vi "MoveToAndRotate.vi"(5 "Camera Offset Y":dbl, 6 "Initial Angle":dbl, 7 "Camera Offset X":dbl, 8 "Error In":errorcluster, 9 "Probing Array":dbl[][](array[numeric]), 10 "Probe Index":i32, 11 "connection ID":refnum<k5>) -> (0 "error out":errorcluster, 3 "connection ID 2":refnum<k5>)   [LabVIEW 2018]
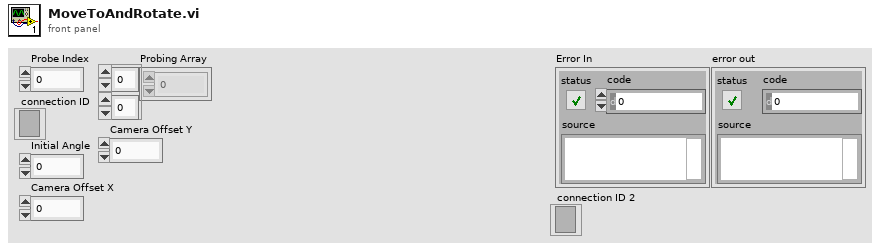
[diagram p1: front panel]
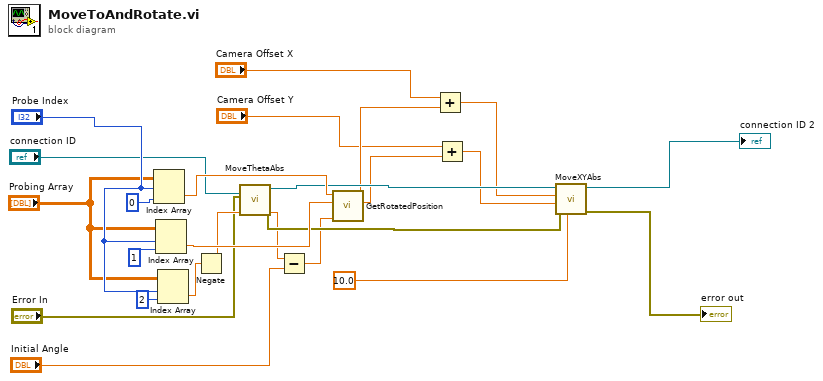
[diagram p0: block diagram]
diagram:
  n1 = Index Array(array="Probing Array", index (row)="Probe Index", index (col)=0 ("index")) -> (element=w21:dbl)
  n2 = Index Array(array="Probing Array", index (row)="Probe Index", index (col)=1 ("index")) -> (element=w22:dbl)
  n3 = Index Array(array="Probing Array", index (row)="Probe Index", index (col)=2 ("disabled index (col)")) -> (element=w15:dbl)
  n4 = Negate(x=w15) -> (-x=w18:dbl)
  n5 = call "MoveThetaAbs.vi"("Theta"=w18, "error out 2"="Error In", "connection ID"="connection ID") -> ("ThetaOut (rad)"=w14:dbl, "error out"=w19:errorcluster, "connection ID 2"=w20:refnum<k5>)  [unwired: 6 in]
  n6 = Subtract(x=w14, y="Initial Angle") -> (x-y=w13:dbl)
  n7 = call "GetRotatedPosition.vi"("theta"=w13, "Y"=w22, "X"=w21) -> ("Y'"=w6:dbl, "X'"=w5:dbl)  [unwired: 7 in]
  n8 = Add(x="Camera Offset X", y=w5) -> (x+y=w3:dbl)
  n9 = Add(x="Camera Offset Y", y=w6) -> (x+y=w4:dbl)
  n10 = call "MoveXYAbs.vi"("%Speed"=10.0, "error in (no error) 2"=w19, "Y"=w4, "X"=w3, "connection ID 2"=w20) -> ("error out"=→"error out":errorcluster, "connection ID"=→"connection ID 2":refnum<k5>)  [unwired: 5 in]
